vi "Teleop.vi"(10 "Match Info":T1={"Autonomous Elapsed Seconds"=0.0, "TeleOp Elapsed Seconds"=0.0, "Disabled Elapsed Seconds"=0.0, "Visited Autonomous"=FALSE, "Visited TeleOp"=FALSE, "Visited Disabled"=FALSE, "Autonomous Settings"={"Autonomous Style"=enum."Independent", "VI Refnum"=refnum}}, 11 "Call Context":T2) -> ()   [LabVIEW 2014]
doc: "This VI is called for each TeleOp packet received from the DS where the robot is not disabled. It is often used to read from the joysticks and update I/O or to update setpoints for timed control loops. It should complete and return within 20 milliseconds or it may miss DS packets."
uses:
  <vilib>/Rock Robotics/WPI/DriverStation/WPI_DriverStationDerivedRobotMode.ctl
  <vilib>/Rock Robotics/WPI/DriverStation/WPI_DriverStationMatch Info.ctl
  <vilib>/Rock Robotics/WPI/RobotDrive/WPI_RobotDriveGetSetRefNum.vi
  <vilib>/Rock Robotics/WPI/Joystick/WPI_JoystickGetSetRefNum.vi
  Robot Global Data.vi
panel:
  out "Sample Boolean 1":bool
  out "Sample Boolean 0":bool
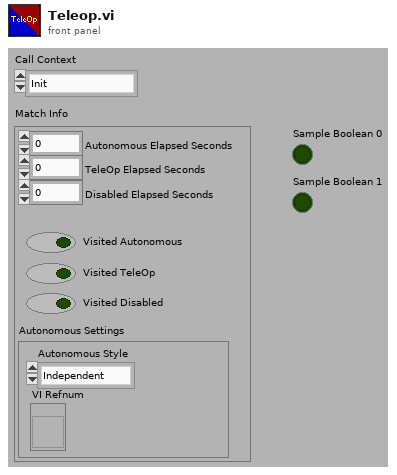
[diagram p1: front panel]
types:
  T1 = typedef "WPI_DriverStationMatch Info.ctl" = cluster{"Autonomous Elapsed Seconds":dbl, "TeleOp Elapsed Seconds":dbl, "Disabled Elapsed Seconds":dbl, "Visited Autonomous":bool, "Visited TeleOp":bool, "Visited Disabled":bool, "Autonomous Settings":cluster{"Autonomous Style":enum16{"Iterative", "Independent"}, "VI Refnum":refnum<vi>}}
  T2 = typedef "WPI_DriverStationDerivedRobotMode.ctl" = enum16{"Init", "Execute", "Stop"}
  T3 = typedef "WPI_RobotDriveDevRef.ctl" = cluster{"DevStatus":errorcluster, "Motors[]":T4[], "Square Inputs":bool, "Max Output":dbl}
  T4 = typedef "WPI_MotorControlDeviceRef.ctl" = cluster{"DeviceStatus":errorcluster, "Type":enum16{"PWM", "CAN"}, "PWM":cluster{"Digital Module":T5, "PWM Channel":T6, "DeadBand":T7}, "CAN":cluster{"Device Number":u8, "Control Mode":T8, "Semaphore":T9, "Max Vout":dbl}, "Invert":bool, "TransformRef":T10, "InvTransformRef":T10}
  T5 = typedef "FPGA_TypedefDigitalModule.ctl" = enum16{"Digital Module 1", "Digital Module 2"}
  T6 = typedef "FPGA_DIOPWMChannel.ctl" = enum8{"PWM 1", "PWM 2", "PWM 3", "PWM 4", "PWM 5", "PWM 6", "PWM 7", "PWM 8", "PWM 9", "PWM 10", "Invalid"}
  T7 = typedef "WPI_PWMDeadband.ctl" = cluster{"Name":string, "maxPositivePwm":i32, "minPositivePwm":i32, "centerPwm":i32, "maxNegativePwm":i32, "minNegativePwm":i32, "angularRange":u16}
  T8 = typedef "WPI_CANJaguar_ControlMode.ctl" = enum8{"Percent VBus", "Current", "Speed", "Position", "Voltage"}
  T9 = typedef "Semaphore RefNum" = refnum<k1>
  T10 = typedef "WPI_PWMTransform_ConPane.ctl" = refnum<vi>
  T11 = typedef "WPI_JoystickDevRef.ctl" = cluster{"Device":T12}
  T12 = typedef "WPI_JoystickDeviceEnum.ctl" = enum16{"USB 0", "USB 1", "USB 2", "USB 3", "USB 4", "USB 5"}
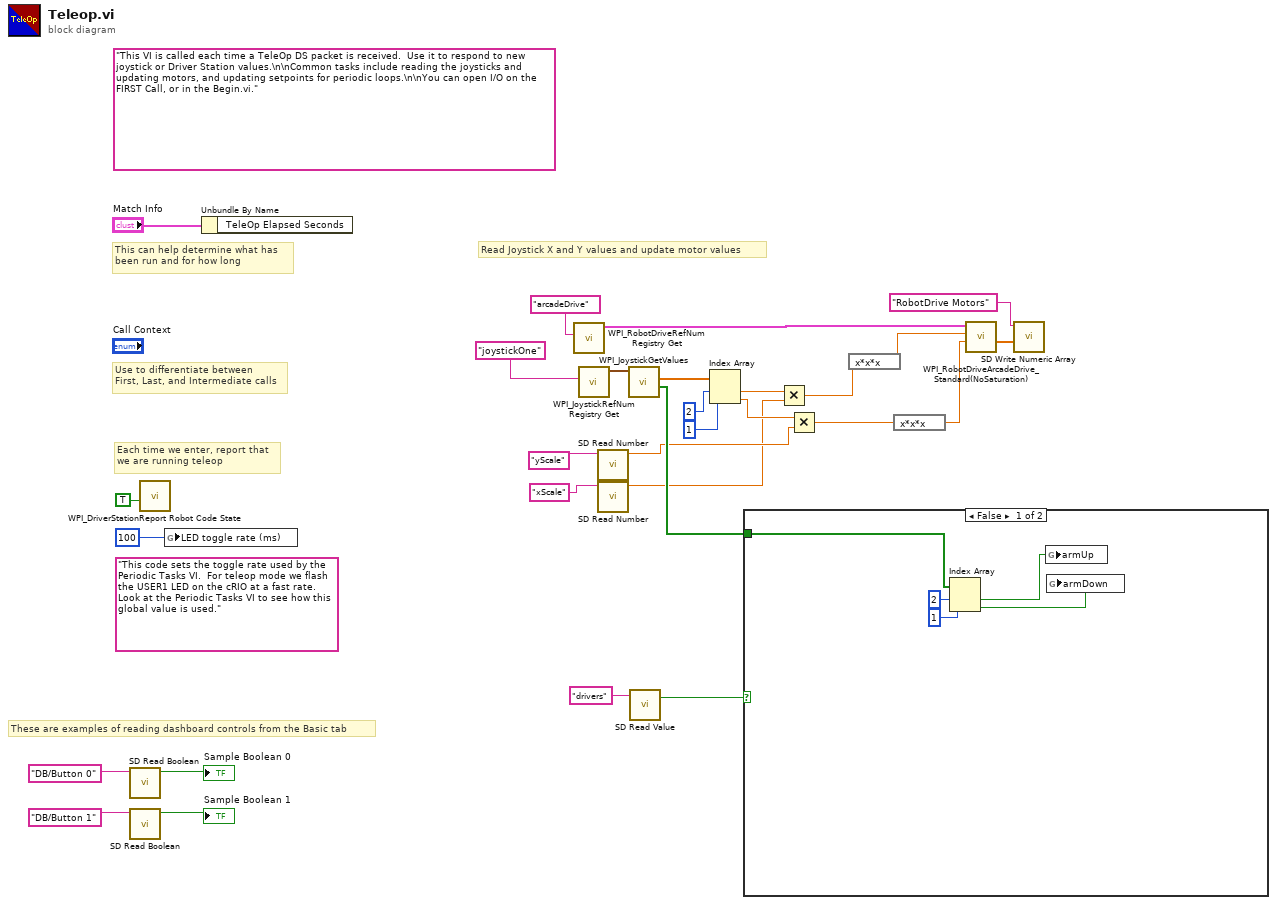
[diagram p0: block diagram]
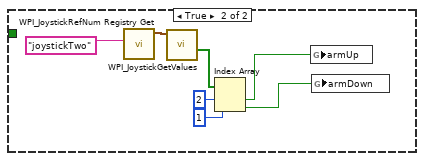
[diagram p2: hidden frame]
diagram:
  (unwired) "This code sets the toggle rate used by the Periodic Tasks VI.  For teleop mode we flash the USER1 LED on the cRIO at a fast rate.  Look at the Periodic Tasks VI to see how this global value is used."
  (unwired) "This VI is called each time a TeleOp DS packet is received.  Use it to respond to new joystick or Driver Station values.\n\nCommon tasks include reading the joysticks and updating motors, and updating setpoints for periodic loops.\n\nYou can open I/O on the FIRST Call, or in the Begin.vi."
  # "These are examples of reading dashboard controls from the Basic tab"
  # "Each time we enter, report that\nwe are running teleop"
  # "Use to differentiate between\nFirst, Last, and Intermediate calls"
  # "This can help determine what has\nbeen run and for how long"
  # "Read Joystick X and Y values and update motor values"
  n1 = call <vilib>:"SD Read Boolean.vi"("Name"="DB/Button 0" ("refnum name")) -> ("Boolean"=→"Sample Boolean 0":bool)  [unwired: 8 in, 2 out]
  n2 = call <vilib>:"SD Read Boolean.vi"("Name"="DB/Button 1" ("refnum name")) -> ("Boolean"=→"Sample Boolean 1":bool)  [unwired: 8 in, 2 out]
  n3 = call <vilib>:"WPI_DriverStationReport Robot Code State.vi"("TeleOp"=TRUE ("Autonomous")) -> ()  [unwired: 10 in, 1 out]
  n4 = global write "Robot Global Data.vi" "LED toggle rate (ms)"(u32 100 ("LED ms toggle rate")) -> ()
  n5 = Unbundle By Name("Match Info") -> ()  [unwired: 1 out]
  n6 = call <vilib>:"WPI_RobotDriveRefNum Registry Get.vi"("refnum name"="arcadeDrive") -> ("RobotDriveDevRef"=w27:T3)  [unwired: 1 in, 9 out]
  n7 = call <vilib>:"WPI_JoystickRefNum Registry Get.vi"("refnum name"="joystickOne") -> ("JoystickDevRef"=w25:T11)  [unwired: 1 in, 9 out]
  n8 = call <vilib>:"SD Read Number.vi"("Name"="yScale" ("refnum name")) -> ("Numeric"=w9:dbl)  [unwired: 8 in, 2 out]
  n9 = call <vilib>:"SD Read Number.vi"("Name"="xScale" ("refnum name")) -> ("Numeric"=w3:dbl)  [unwired: 8 in, 2 out]
  n10 = call <vilib>:"WPI_JoystickGetValues.vi"("JoystickDevRef"=w25) -> ("Buttons"=w12:bool[], "Axes"=w15:dbl[])  [unwired: 6 in, 3 out]
  n11 = call-poly <vilib>:"SD Read Value.vi"("Name"="drivers") -> ("Boolean"=w13:bool)  [unwired: 8 in, 2 out]
  n12 = Index Array(array=w15, index #1=2 ("index"), index #2=1 ("index")) -> (element #1=w8:dbl, element #2=w10:dbl)
  n13 = case shown="False" w13 {
    tunnel: w12 -> [w32 _]
    frame False {
      n14 = Index Array(array=w32, index #1=2 ("index"), index #2=1 ("index")) -> (element #1=w31:bool, element #2=w30:bool)
      n15 = global write "Robot Global Data.vi" "armUp"(w31) -> ()
      n16 = global write "Robot Global Data.vi" "armDown"(w30) -> ()
    }
    frame True {
      n17 = call <vilib>:"WPI_JoystickRefNum Registry Get.vi"("refnum name"="joystickTwo") -> ("JoystickDevRef"=w38:T11)  [unwired: 1 in, 9 out]
      n18 = call <vilib>:"WPI_JoystickGetValues.vi"("JoystickDevRef"=w38) -> ("Buttons"=w39:bool[])  [unwired: 6 in, 4 out]
      n19 = Index Array(array=w39, index #1=2 ("index"), index #2=1 ("index")) -> (element #1=w36:bool, element #2=w35:bool)
      n20 = global write "Robot Global Data.vi" "armUp"(w36) -> ()
      n21 = global write "Robot Global Data.vi" "armDown"(w35) -> ()
    }
  }
  n22 = Multiply(x=w8, y=w3) -> (x*y=w4:dbl)
  n23 = Multiply(x=w10, y=w9) -> (x*y=w11:dbl)
  n24 = expression code="x*x*x"(w4) -> (w1:dbl)
  n25 = expression code="x*x*x"(w11) -> (w2:dbl)
  n26 = call <vilib>:"WPI_RobotDriveArcadeDrive_Standard(NoSaturation).vi"("Y axis value"=w2, "X axis value"=w1, "RobotDriveDevRef"=w27) -> ("Motor Values"=w21:dbl[])  [unwired: 1 in, 7 out]
  n27 = call <vilib>:"SD Write Numeric Array.vi"("Numeric Array"=w21, "Name"="RobotDrive Motors") -> ()  [unwired: 8 in, 2 out]
